vi "Export.vi"(8 "error in":errorcluster, 11 "Objects":T1) -> (0 "error out":errorcluster)   [LabVIEW 2017, in "J1939 editor node.lvclass"]
uses:
  J1939 editor node.lvclass
  <vilib>/NI/DCAF/Tag Editor Core/Table API/Table Manager/object ref.ctl
  <vilib>/NI/DCAF/Tag Editor Core/Configuration Editor/Classes/Engine Parent/Engine Parent Editor Node.lvclass
  <vilib>/NI/DCAF/Tag Editor Core/Configuration Editor/Classes/Module editor node/module editor node.lvclass
  <vilib>/NI/DCAF/Tag Editor Core/Table API/Table Manager/Table Manager.lvclass
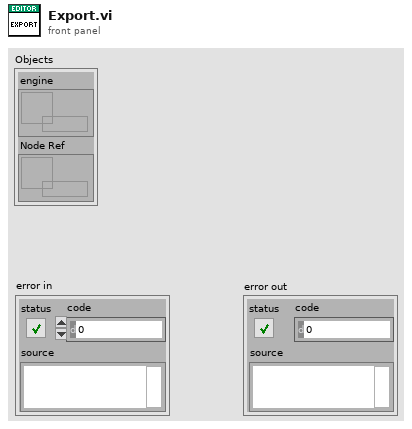
[diagram p1: front panel]
types:
  T1 = typedef "Table Manager.lvlib/Table Manager.lvclass/object ref.ctl" = cluster{"engine":refnum<data-value>, "Node Ref":refnum<data-value>}
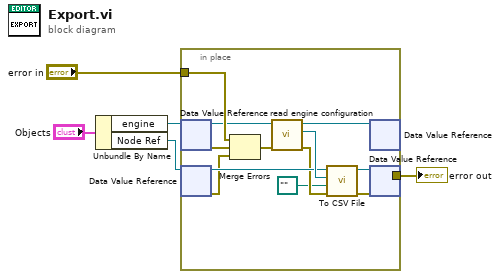
[diagram p0: block diagram]
diagram:
  n1 = Unbundle By Name("Objects") -> ("engine"=w2:refnum<data-value>, "Node Ref"=w1:refnum<data-value>)
  n2 = in-place {
    in-place-border: "error in" -> [w17]
    in-place-border: [w12] -> w3
    n3 = in-place-dvr #1(w2) -> (w16:refnum<class "Engine Parent Editor Node.lvclass">, w8:errorcluster)
    n4 = in-place-dvr #2(w1) -> (w14:refnum<class "module editor node.lvclass">, w7:errorcluster)
    n5 = Merge Errors(w17, w8, w7) -> (w11:errorcluster)
    n6 = call <vilib>:"read engine configuration.vi"("error in"=w11, "Engine Parent Editor Node in"=w16) -> ("error out"=w10:errorcluster, "engine configuration"=w15:refnum<class "engine configuration.lvclass">, "Engine Parent Editor Node out"=w9:refnum<class "Engine Parent Editor Node.lvclass">)  [unwired: 7 in]
    n7 = call-dynamic "To CSV File.vi"("error in (no error)"=w10, "Path"=path "", "engine configuration"=w15, "module editor node in"=w14) -> ("error out"=w12:errorcluster, "module editor node out"=w13:refnum<class "module editor node.lvclass">)  [unwired: 6 in]
    n8 = in-place-dvr #1(w9) -> ()  [unwired: 2 out]
    n9 = in-place-dvr #2(w13) -> ()  [unwired: 2 out]
  }
  "error out" <- w3
